vi "Read longname.vi"(8 "error in (no error)":errorcluster, 11 "file attributes in":refnum<class "File Attributes.lvclass">) -> (0 "error out":errorcluster, 2 "long name":string, 3 "file attributes out":refnum<class "File Attributes.lvclass">)   [LabVIEW 2020, in "NI_SFTP.lvlib" / "File Attributes.lvclass"]
doc: "Reads the long listing of this File Attributes object. The contents of this listing is server-dependent.\n\nThe long listing is a server-generated string analogous to the output of the `ls -l` output on a Unix system. The long listing may be used to summarize remote file information such as size and permissions.\n\nLong listings may contain symbolic ownership information. However, the SFTP protocol itself does not support symbolic itself.\n\nThis property may not always be populated by SFTP VIs. If it does not exist, an error is returned."
uses:
  <vilib>/net/SFTP/File Attributes/File Attributes.lvclass
  <vilib>/net/SFTP/File Attributes/File Attributes.lvclass/File Attributes.ctl
  <vilib>/Utility/error.llb/Error Cluster From Error Code.vi
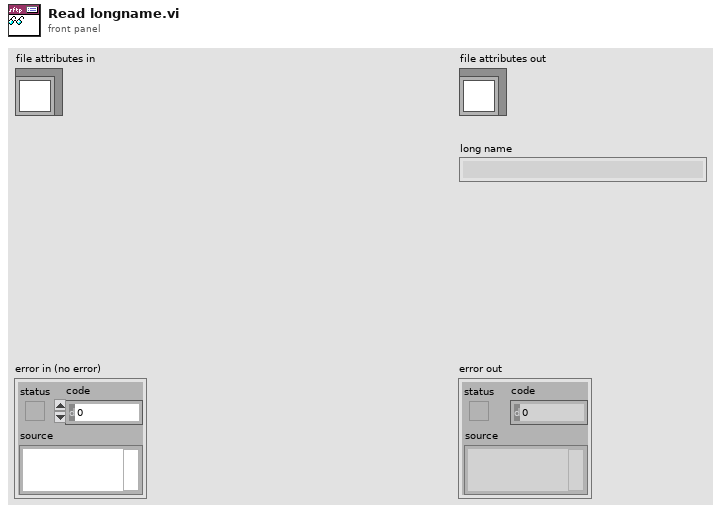
[diagram p1: front panel]
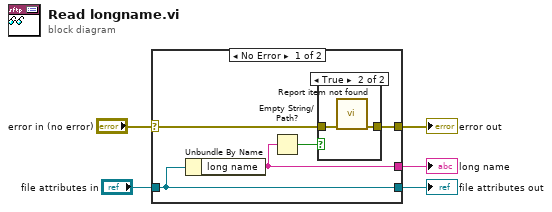
[diagram p0: block diagram]
diagram:
  n1 = case shown="No Error" "error in (no error)" {
    selector: "error in (no error)" -> [w7 w14]
    tunnel: [w10 w15] -> w2
    tunnel: "file attributes in" -> [w10 w15]
    tunnel: [w9 _] -> w1
    tunnel: [w6 w14] -> w3
    frame No Error {
      n2 = Unbundle By Name(w10) -> ("long name"=w9:string)
      n3 = Empty String/Path?(string/path=w9) -> (empty?=w8:bool)
      n4 = case shown="True" w8 {
        tunnel: w7 -> [w11 w13]
        tunnel: [w11 w12] -> w6
        frame False {
        }
        frame True {
          n5 = call <vilib>:"Report item not found.vi"("error in (no error)"=w13) -> ("error out"=w12:errorcluster)  [unwired: 10 in]
        }
      }
    }
    frame Error {
    }
  }
  "error out" <- w3
  "file attributes out" <- w2
  "long name" <- w1
